vi "countrate.vi"() -> ()   [LabVIEW 2015]
uses:
  <vilib>/Platform/TimedLoop/XDataNode/timing_clust.ctl
  <vilib>/Platform/TimedLoop/XDataNode/nitl_modes.ctl
  <vilib>/Platform/TimedLoop/XDataNode/wakeup.ctl
  <vilib>/Utility/file.llb/Write Delimited Spreadsheet (I64).vi
  <vilib>/platform/TimedLoop/XDataNode/XDataNode.xnode
  <vilib>/Platform/TimedLoop/XDataNode/XDNodeRunTimeDep.lvlib
panel:
  out "XY Graph":cluster{i32, i32}[](graph)
  out "Numeric":i32=9
  in  "Total Time":dbl=120.0
  in  "file path (dialog if empty)":path
  in  "Period":i64=1
  out "counts per second":dbl(knob)=57.0 scale=0.0..100.0
  in  "stop":bool
  # "Demo count rate VI for Physics 434"
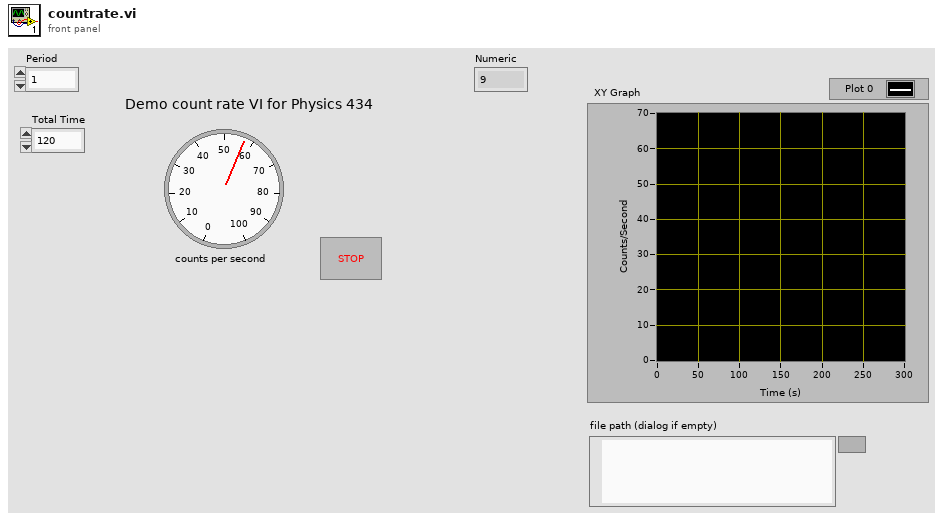
[diagram p1: front panel]
types:
  T1 = typedef "XDNodeRunTimeDep.lvlib/timing_clust.ctl" = cluster{"Expected End [f-1]":u64, "Actual End [f-1]":u64, "Finished Late? [f-1]":bool, "Expected End [i-1]":u64, "Actual End [i-1]":u64, "Finished Late? [i-1]":bool, "Expected Start [i]":u64, "Actual Start [i]":u64, "Expected Start [f]":u64, "Actual Start [f]":u64, "Source Name":string, "Structure Name":string, "Period":i64, "Deadline":i64, "Offset":i64, "Start":i64, "Priority":i32, "Timeout":i32, "Mode":T2, "Wakeup Reason":T3, "Error":errorcluster, "Source Type":string, "Secondary Source Type":string, "Global End Time":u64, "Global Start Time":u64, "Frame Duration":u64, "Iteration Duration":u64, "Assigned CPU":i32, "I/O Scan Engine Mode":u32}
  T2 = typedef "XDNodeRunTimeDep.lvlib/nitl_modes.ctl" = enum32{"No Change", "Process missed periods, maintain original phase", "Discard missed periods, maintain original phase", "Process missed periods, ignore original phase", "Discard missed periods, ignore original phase"}
  T3 = typedef "XDNodeRunTimeDep.lvlib/wakeup.ctl" = enum32{"Normal", "Aborted", "Asynchronous wakeup", "Timing source error", "Timed loop error", "Timeout"}
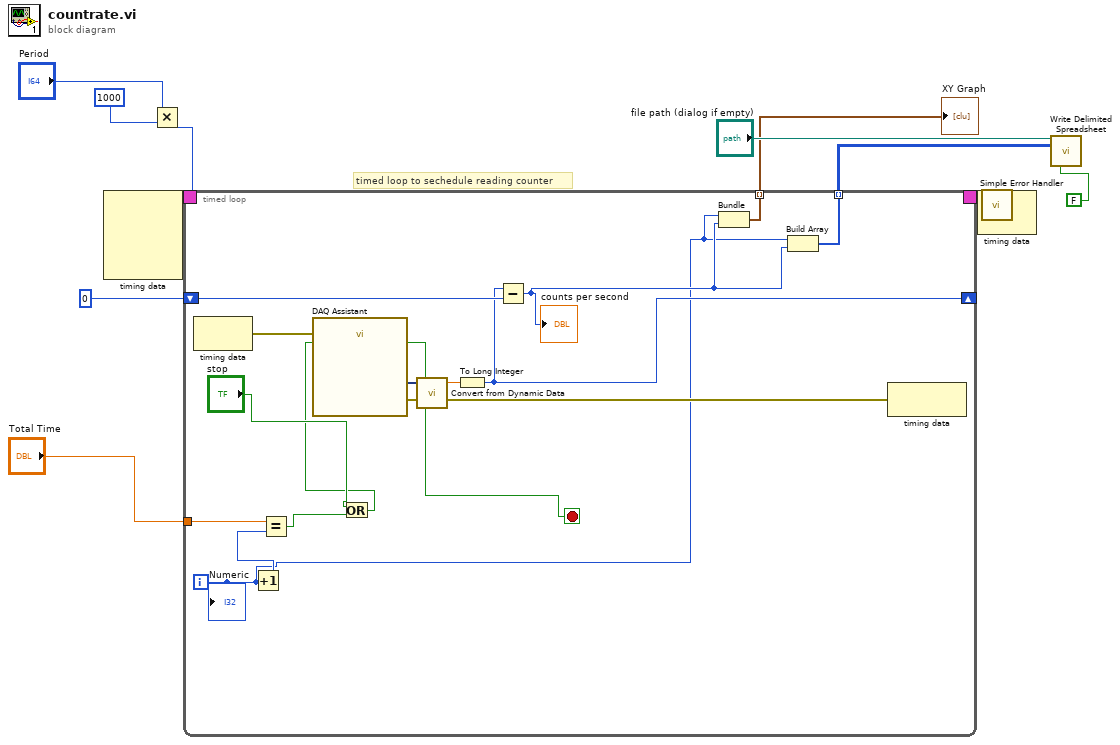
[diagram p0: block diagram]
diagram:
  # "timed loop to sechedule reading counter"
  n1 = Multiply(x="Period", y=i64 1000) -> (x*y=w4:i64)
  n2 = node-c288(w4) -> (w12:T1)  [unwired: 3 in]
  n3 = timed-loop {
    timing: w12 -> [_]
    timing-out: [_] -> w11
    shift-right: [w26] -> _
    shift-left: 0 -> [w27]
    tunnel: "Total Time" -> [w22]
    tunnel: [w17] -> w2 mode=indexing
    tunnel: [w14] -> w1 mode=indexing
    i -> [w13]
    stop <- w20 stop-if-true
    n4 = node-c288() -> (w23:errorcluster)  [unwired: 1 in]
    n5 = Increment(x=w13) -> (x+1=w16:i32)
    n6 = Equal?(x=w22, y=w16) -> (x = y?=w21:bool)
    n7 = Or(x="stop", y=w21) -> (x .or. y?=w18:bool)
    n8 = call "DAQ Assistant"("error in"=w23, "stop (F)"=w18) -> ("data"=w28:dynamicdata, "stopped"=w20:bool, "error out"=w24:errorcluster)  [unwired: 14 in, 1 out]
    n9 = call "Convert from Dynamic Data"("Dynamic Data Type"=w28) -> ("Scalar"=w25:dbl)  [unwired: 3 in]
    n10 = To Long Integer(number=w25) -> (32bit integer=w26:i32)
    n11 = Subtract(x=w26, y=w27) -> (x-y=w15:i32)
    "counts per second" <- w15
    n12 = Bundle(w13, w15) -> (w14:cluster{i32, i32})  [unwired: 1 in]
    n13 = Build Array(w13, w15) -> (w17:i32[])
    n14 = node-c288(w24) -> ()  [unwired: 1 out]
    "Numeric" <- w13
  }
  "XY Graph" <- w1
  n15 = node-c288(w11) -> (w9:errorcluster)
  n16 = call <vilib>:"Simple Error Handler.vi"("error in (no error)"=w9) -> ()  [unwired: 4 in, 5 out]
  n17 = call-poly <vilib>:"Write Delimited Spreadsheet.vi"("file path (dialog if empty)"="file path (dialog if empty)", "2D data"=w2, "transpose? (F)"=FALSE) -> ()  [unwired: 11 in, 2 out]
